vi "Python.vi"() -> ()   [LabVIEW 2014]
uses:
  Controls/Standard Action.ctl
  Controls/StageStates.ctl
  <vilib>/Analysis/baseanly.llb/Mean (DBL).vi
  <vilib>/Analysis/NI_AALBase.lvlib
panel:
  out "queue":string
  out "standard output":string
  out "standard error":string
  out "DM1":dbl[][](graph)
  out "DM0":dbl[][](graph)
  out "Image 2":sgl[][](graph)
  in  "launch_python":bool
  in  "script name":string="sensorless.py"
  in  "arguments":string="--zmin 11 --zmax 12 --nm-maxfev 80 --runs 1 --modes4pi --aberration-rms 0.0 --metric metric_low_spatial_freq modal"
  in  "Run Python":bool
  in  "Exit":bool
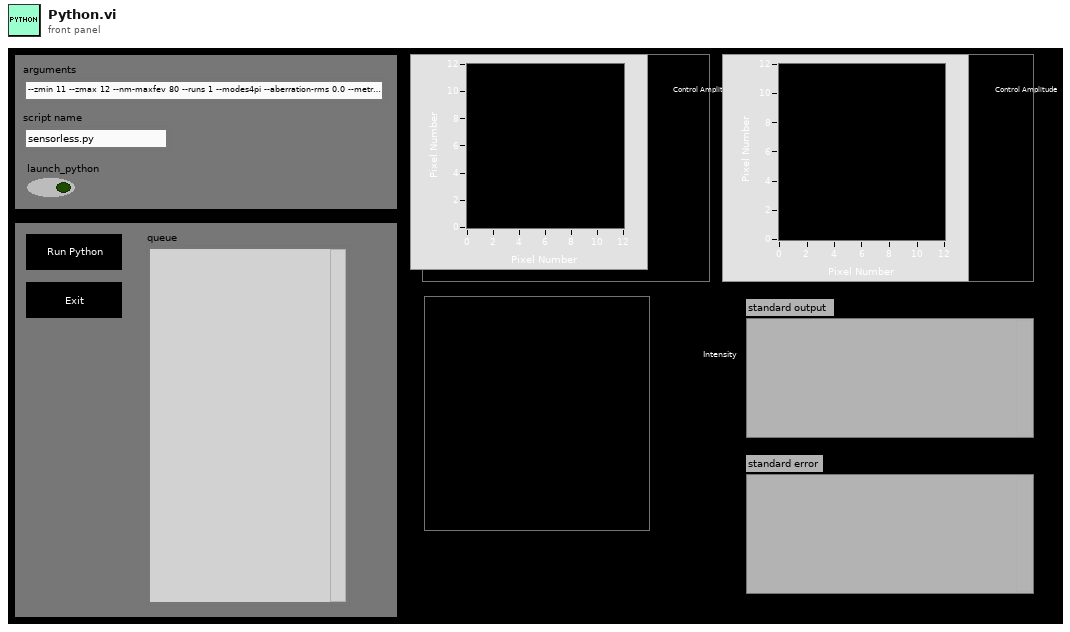
[diagram p1: front panel]
types:
  T1 = typedef "Standard Action.ctl" = enum16{"Read", "Write"}
  T2 = typedef "StageStates.ctl" = enum16{"POSITION", "MVR", "MOVE", "HALT", "ONTARGET", "ERROR", "EXIT", "HOME", "ZEROPOS", "NANOPOS", "QUIT", "ANALOG"}
  T3 = typedef "MirrorModes_DUAL.ctl" = cluster{"Mode":string, "Amplitude":dbl}[][]
  T4 = typedef "Image Acquisition Parameters.ctl" = cluster{"Scan Type":enum16{"Sample Scanning", "Beam Scanning"}, "Scan Mode":enum16{"XY", "XZ", "YZ", "XYZ"}, "Fast Axis Frequency (Hz)":dbl, "Image Format":u16, "Line Accumulations":u16, "Frames Per Capture":u16, "Frames Accumulations":u16, "Image Dimension (um)":dbl[], "Number of Z Steps":u16, "Z Steps Size (um)":dbl, "Pixel Size (nm)":dbl[], "Customized Image Format":dbl[]}
  T5 = typedef "Detectors.ctl" = cluster{"PMT":bool, "Far Red (685/40 nm)":bool, "Orange (624/40 nm)":bool, "Green (525/50 nm)":bool, "Sum All":bool}
  T6 = typedef "Laser Controls.ctl" = cluster{"STED Power (V)":dbl, "STED":bool, "650 nm":bool, "590 nm":bool, "485 nm":bool, "Manual Control":bool}
  T7 = cluster{"dm0":dbl[], "dm1":dbl[], "zcomp":dbl, "stack":sgl[][]}
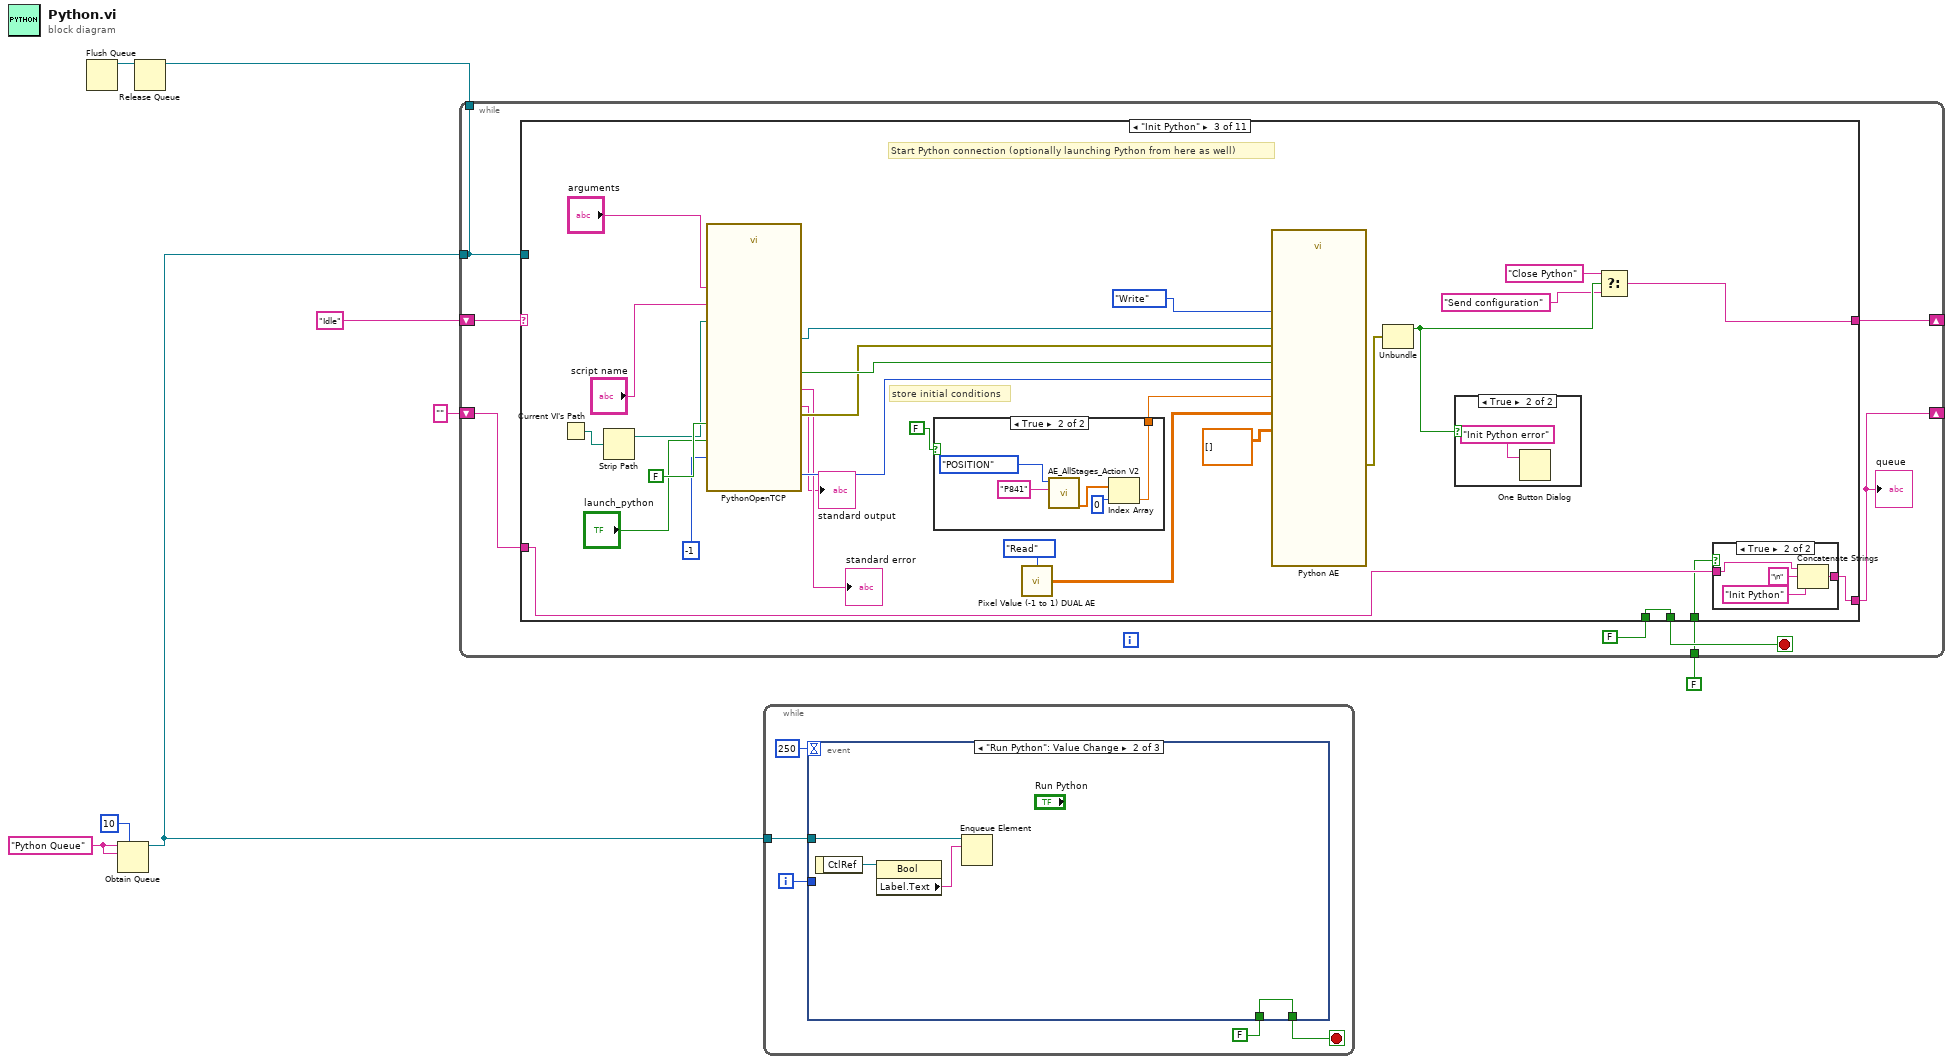
[diagram p0: block diagram]
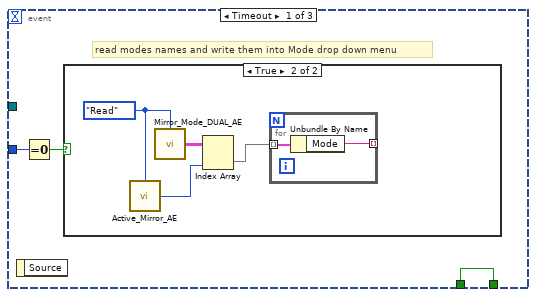
[diagram p2: hidden frame]
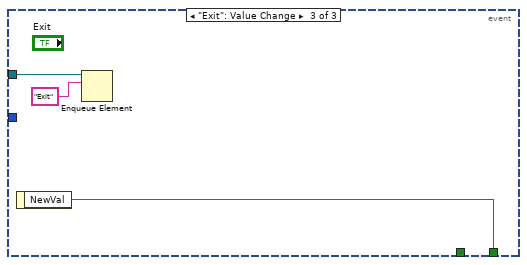
[diagram p4: hidden frame]
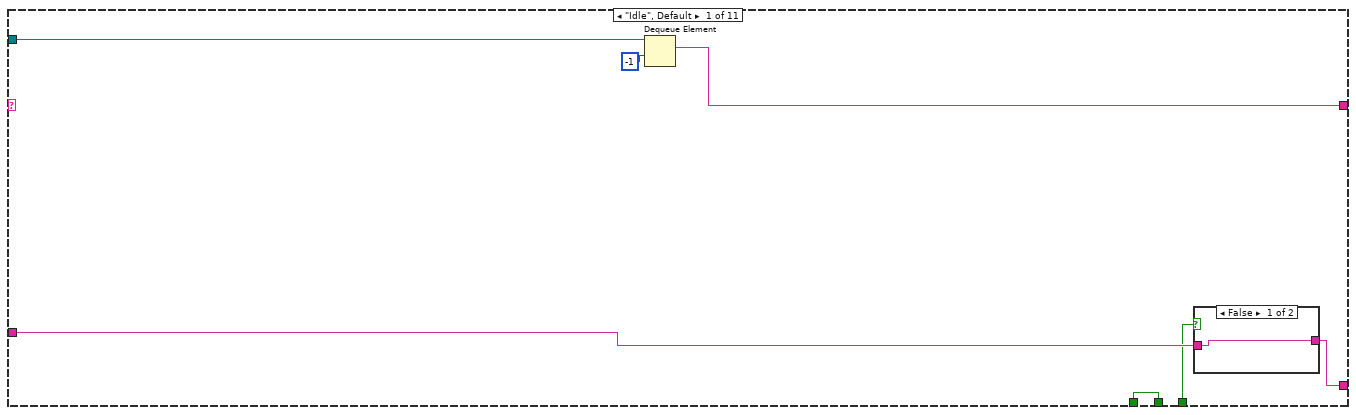
[diagram p5: hidden frame]
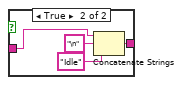
[diagram p6: hidden frame]
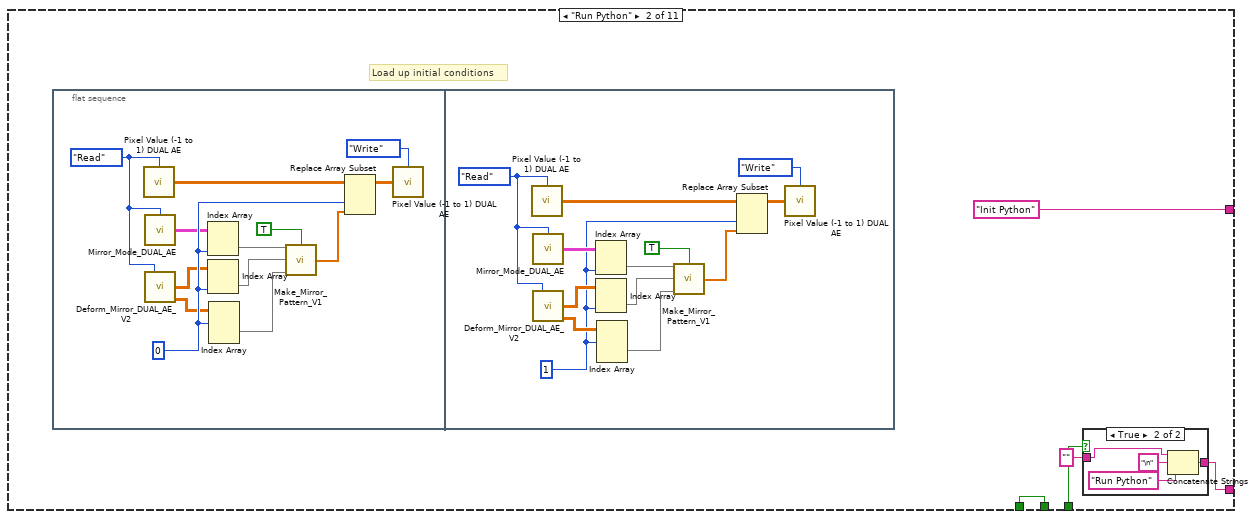
[diagram p7: hidden frame]
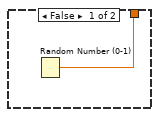
[diagram p10: hidden frame]
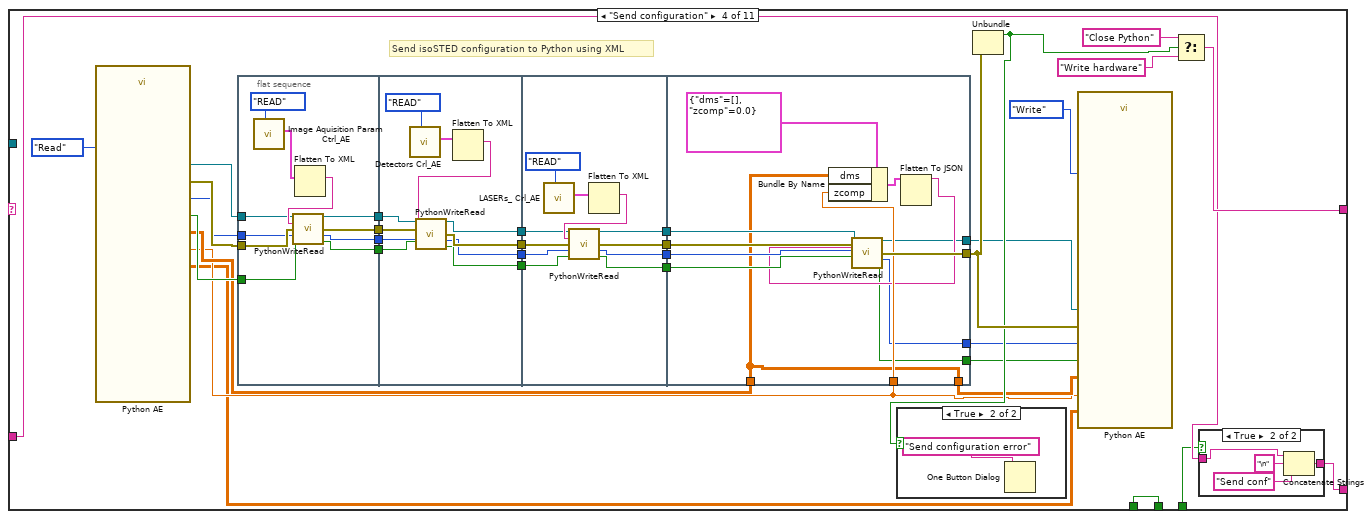
[diagram p12: hidden frame]
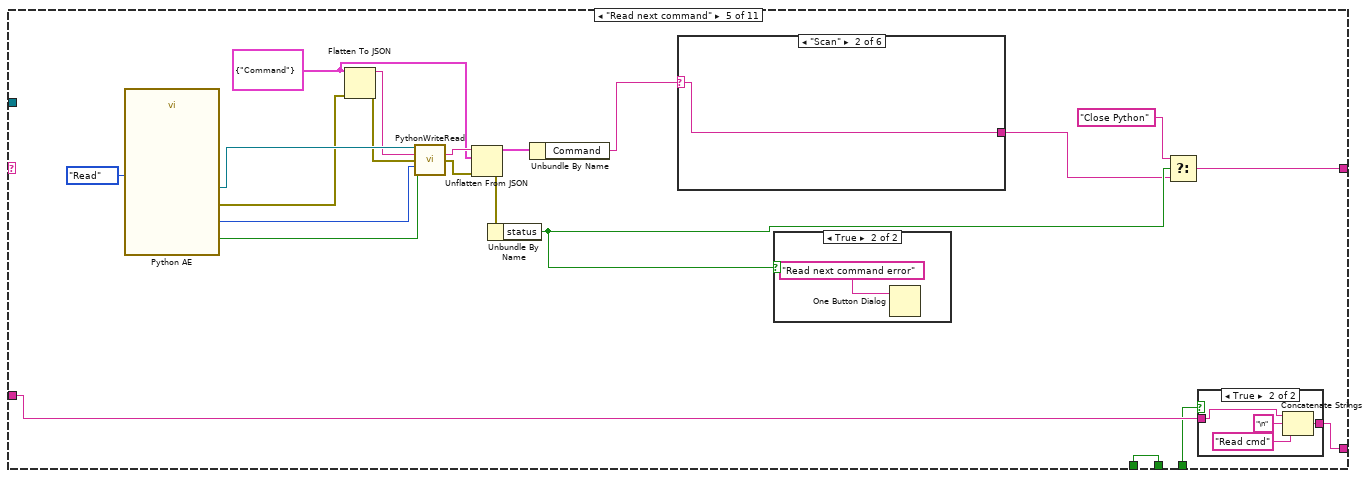
[diagram p15: hidden frame]
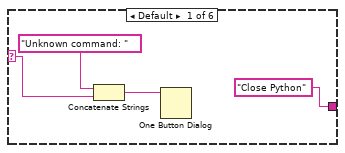
[diagram p17: hidden frame]
diagram:
  w7 = "Python Queue" ("name (unnamed)")
  n1 = Obtain Queue(max queue size (-1, unlimited)=10, name (unnamed)=w7, element data type=w7) -> (queue out=w5:refnum<queue>)  [unwired: 2 in, 2 out]
  n2 = while {
    shift-right: [w11] -> _
    shift-left: "Idle" -> [w13]
    tunnel: w5 -> [w15]
    tunnel: [w15] -> w4
    shift-right: [w10] -> _
    shift-left: "" -> [w12]
    tunnel: FALSE -> [w9]
    stop <- w16 stop-if-true
    n3 = case shown="\"Init Python\"" w13 {
      tunnel: [w20 w33 w82 w119 w210 w247 w270 w331 w364 w433 TRUE] -> w16
      tunnel: w15 -> [w22 _ _ _ _ _ _ _ _ _ _]
      tunnel: [w21 "Init Python" ("name (unnamed)") w70 w116 w195 w231 "Python pipe" ("name (unnamed)") w332 "Read next command" ("name (unnamed)") "Idle" ("name (unnamed)") "Exit" ("name (unnamed)")] -> w11
      tunnel: FALSE -> [w20 w33 w82 w119 w210 w247 w270 w331 w364 w433 _]
      tunnel: w12 -> [w19 _ w67 w107 w193 w228 w254 w318 w357 w420 w441]
      tunnel: [w17 w31 w66 w106 w192 w229 w256 w319 w356 w419 w442] -> w10
      tunnel: w9 -> [w18 w30 w65 w105 w191 w227 w255 w317 w358 w418 w440]
      frame "Idle", Default {
        n4 = Dequeue Element(queue=w22, timeout in ms (-1)=-1) -> (element=w21:string)  [unwired: 1 in, 3 out]
        n5 = case shown="False" w18 {
          tunnel: [w24 w26] -> w17
          tunnel: w19 -> [w24 w25]
          frame False {
          }
          frame True {
            n6 = Concatenate Strings(w25, "\n" ("string"), "Idle" ("string")) -> (w26:string)
          }
        }
      }
      frame "Run Python" {
        # "Load up initial conditions"
        n7 = flat-sequence {
          frame #0 {
            w51 = 0 ("index (col)")
            w47 = Standard_Action."Read" ("Action")
            n8 = call "Pixel Value (-1 to 1) DUAL AE.vi"("Action"=w47) -> ("Pixel Value (-1 to 1) Out"=w48:dbl[][])  [unwired: 14 in]
            n9 = call "Mirror_Mode_DUAL_AE.vi"("Action"=w47) -> ("Mirror Modes Out"=w44:T3)  [unwired: 14 in]
            n10 = call "Deform_Mirror_DUAL_AE_V2.vi"("Action"=w47) -> ("Flat Files Out"=w42:dbl[][], "Mode Matrix Out"=w40:dbl[][][])  [unwired: 10 in, 3 out]
            n11 = Index Array(array=w44, index (col)=w51) -> (element=w45:cluster{"Mode":string, "Amplitude":dbl}[])  [unwired: 1 in]
            n12 = Index Array(array=w42, index (col)=w51) -> (element=w43:dbl[])  [unwired: 1 in]
            n13 = Index Array(array=w40, index (dim 0)=w51) -> (element=w39:dbl[][])  [unwired: 2 in]
            n14 = call "Make_Mirror_Pattern_V1.vi"("Mirror Modes In"=w45, "Flat On?"=TRUE ("Apply Flat"), "Flat File In"=w43, "Mirror Modes Array"=w39) -> ("Pixel Value U (-1 to 1)"=w49:dbl[])  [unwired: 11 in]
            n15 = Replace Array Subset(array=w48, new element=w49, index (col)=w51) -> (w50:dbl[][])  [unwired: 1 in]
            n16 = call "Pixel Value (-1 to 1) DUAL AE.vi"("Action"=Standard_Action."Write", "Pixel Value (-1 to 1)"=w50) -> ()  [unwired: 13 in, 1 out]
          }
          frame #1 {
            w52 = 1 ("index (col)")
            w56 = Standard_Action."Read" ("Action")
            n17 = call "Pixel Value (-1 to 1) DUAL AE.vi"("Action"=w56) -> ("Pixel Value (-1 to 1) Out"=w55:dbl[][])  [unwired: 14 in]
            n18 = call "Mirror_Mode_DUAL_AE.vi"("Action"=w56) -> ("Mirror Modes Out"=w59:T3)  [unwired: 14 in]
            n19 = call "Deform_Mirror_DUAL_AE_V2.vi"("Action"=w56) -> ("Flat Files Out"=w61:dbl[][], "Mode Matrix Out"=w63:dbl[][][])  [unwired: 10 in, 3 out]
            n20 = Index Array(array=w59, index (col)=w52) -> (element=w58:cluster{"Mode":string, "Amplitude":dbl}[])  [unwired: 1 in]
            n21 = Index Array(array=w61, index (col)=w52) -> (element=w60:dbl[])  [unwired: 1 in]
            n22 = Index Array(array=w63, index (dim 0)=w52) -> (element=w64:dbl[][])  [unwired: 2 in]
            n23 = call "Make_Mirror_Pattern_V1.vi"("Mirror Modes In"=w58, "Flat On?"=TRUE ("Apply Flat"), "Flat File In"=w60, "Mirror Modes Array"=w64) -> ("Pixel Value U (-1 to 1)"=w54:dbl[])  [unwired: 11 in]
            n24 = Replace Array Subset(array=w55, new element=w54, index (col)=w52) -> (w53:dbl[][])  [unwired: 1 in]
            n25 = call "Pixel Value (-1 to 1) DUAL AE.vi"("Action"=Standard_Action."Write", "Pixel Value (-1 to 1)"=w53) -> ()  [unwired: 13 in, 1 out]
          }
        }
        n26 = case shown="True" w30 {
          tunnel: [w34 w36] -> w31
          tunnel: "" -> [w34 w35]
          frame False {
          }
          frame True {
            n27 = Concatenate Strings(w35, "\n" ("string"), "Run Python" ("string")) -> (w36:string)
          }
        }
      }
      frame "Init Python" {
        # "store initial conditions"
        # "Start Python connection (optionally launching Python from here as well)"
        n28 = Current VI's Path() -> (path=w74:path)
        n29 = Strip Path(path=w74) -> (stripped path=w73:path)  [unwired: 1 out]
        n30 = call "PythonOpenTCP.vi"("directory"=w73, "debug"=FALSE, "script name"="script name", "launch_python"="launch_python", "timeout in"=-1 ("timeout ms (60000)"), "arguments"="arguments") -> ("error out"=w83:errorcluster, "connection out"=w86:refnum<k5>, "standard error"=→"standard error":string, "timeout out"=w84:i32, "run_tcp"=w85:bool, "standard output"=→"standard output":string)  [unwired: 4 in]
        n31 = case shown="True" FALSE {
          tunnel: [w98 w99] -> w77
          frame False {
            n32 = Random Number (0-1)() -> (number: 0 to 1=w98:dbl)
          }
          frame True {
            n33 = call "AE_AllStages_Action V2.vi"("Stage ID"="P841" ("StageID"), "Action"=StageStates."POSITION") -> ("Position Out"=w102:dbl[])  [unwired: 7 in, 2 out]
            n34 = Index Array(array=w102, index=0) -> (element=w99:dbl)
          }
        }
        n35 = call "Pixel Value (-1 to 1) DUAL AE.vi"("Action"=Standard_Action."Read") -> ("Pixel Value (-1 to 1) Out"=w80:dbl[][])  [unwired: 14 in]
        n36 = call "Python AE.vi"("connection"=w86, "error"=w83, "run_tcp"=w85, "timeout"=w84, "u"=w80, "zcomp"=w77, "Action"=Standard_Action."Write", "stack"=sgl[][] []) -> ("error out"=w79:errorcluster)  [unwired: 5 in, 6 out]
        n37 = Unbundle(w79) -> ("status"=w72:bool)  [unwired: 2 out]
        n38 = case shown="True" w72 {
          frame False {
          }
          frame True {
            n39 = One Button Dialog(message="Init Python error") -> ()  [unwired: 1 in, 1 out]
          }
        }
        n40 = Select(t="Close Python", s=w72, f="Send configuration" ("name (unnamed)")) -> (s? t:f=w70:string)
        n41 = case shown="True" w65 {
          tunnel: [w93 w95] -> w66
          tunnel: w67 -> [w93 w94]
          frame False {
          }
          frame True {
            n42 = Concatenate Strings(w94, "\n" ("string"), "Init Python" ("string")) -> (w95:string)
          }
        }
      }
      frame "Send configuration" {
        # "Send isoSTED configuration to Python using XML"
        n43 = call "Python AE.vi"("Action"=Standard_Action."Read") -> ("zcomp out"=w109:dbl, "stack out"=w108:sgl[][], "connection out"=w125:refnum<k5>, "error out"=w124:errorcluster, "u out"=w111:dbl[][], "run_tcp out"=w122:bool, "timeout out"=w123:i32)  [unwired: 12 in]
        n44 = flat-sequence {
          tunnel: [w152] -> w138
          tunnel: [w151] -> w137
          tunnel: [w150] -> w136
          tunnel: [w149] -> w135
          tunnel: w125 -> [w148]
          tunnel: w124 -> [w147]
          tunnel: w123 -> [w146]
          tunnel: w122 -> [w145]
          tunnel: w138 -> [w163]
          tunnel: w137 -> [w162]
          tunnel: w136 -> [w161]
          tunnel: w135 -> [w160]
          tunnel: [w159] -> w134
          tunnel: [w158] -> w133
          tunnel: [w157] -> w132
          tunnel: [w156] -> w131
          tunnel: w134 -> [w174]
          tunnel: w133 -> [w173]
          tunnel: w132 -> [w172]
          tunnel: w131 -> [w171]
          tunnel: [w170] -> w130
          tunnel: [w169] -> w129
          tunnel: [w168] -> w128
          tunnel: [w167] -> w127
          tunnel: w130 -> [w189]
          tunnel: w129 -> [w188]
          tunnel: w128 -> [w187]
          tunnel: w127 -> [w186]
          tunnel: [w185] -> w120
          tunnel: w111 -> [w178]
          tunnel: w109 -> [w184]
          tunnel: [w181] -> w114
          tunnel: [w180] -> w113
          tunnel: [w179] -> w112
          tunnel: [w178] -> w110
          frame #0 {
            n45 = call "Image Aquisition Param Ctrl_AE.vi"("Action"=enum16{"READ", "WRITE"}."READ") -> ("Image Acquisition Parameters Out"=w155:T4)  [unwired: 10 in]
            n46 = Flatten To XML(anything=w155) -> (xml string=w153:string)
            n47 = call "PythonWriteRead.vi"("connection in"=w148, "string in"=w153, "error in"=w147, "timeout in"=w146, "run_tcp in"=w145) -> ("connection out"=w152:refnum<k5>, "error out"=w151:errorcluster, "timeout out"=w150:i32, "run_tcp out"=w149:bool)  [unwired: 6 in, 1 out]
          }
          frame #1 {
            n48 = call "Detectors Crl_AE.vi"("Action"=enum16{"READ", "WRITE"}."READ") -> ("Detectors Parameters Out"=w165:T5)  [unwired: 10 in]
            n49 = Flatten To XML(anything=w165) -> (xml string=w164:string)
            n50 = call "PythonWriteRead.vi"("connection in"=w163, "string in"=w164, "error in"=w162, "timeout in"=w161, "run_tcp in"=w160) -> ("connection out"=w159:refnum<k5>, "error out"=w158:errorcluster, "timeout out"=w157:i32, "run_tcp out"=w156:bool)  [unwired: 6 in, 1 out]
          }
          frame #2 {
            n51 = call "LASERs_ Crl_AE.vi"("Action"=enum16{"READ", "WRITE"}."READ") -> ("Laser Parameters Out"=w177:T6)  [unwired: 10 in]
            n52 = Flatten To XML(anything=w177) -> (xml string=w175:string)
            n53 = call "PythonWriteRead.vi"("connection in"=w174, "string in"=w175, "error in"=w173, "timeout in"=w172, "run_tcp in"=w171) -> ("connection out"=w170:refnum<k5>, "error out"=w169:errorcluster, "timeout out"=w168:i32, "run_tcp out"=w167:bool)  [unwired: 6 in, 1 out]
          }
          frame #3 {
            n54 = Bundle By Name(cluster=cluster{"dms":dbl[][], "zcomp":dbl} {"dms"=[], "zcomp"=0.0} ("input cluster"), "dms"=w178, "zcomp"=w184) -> (w183:cluster{"dms":dbl[][], "zcomp":dbl})
            n55 = Flatten To JSON(anything=w183) -> (JSON string=w182:string)  [unwired: 2 in, 1 out]
            n56 = call "PythonWriteRead.vi"("connection in"=w189, "string in"=w182, "error in"=w188, "timeout in"=w187, "run_tcp in"=w186) -> ("connection out"=w181:refnum<k5>, "error out"=w185:errorcluster, "timeout out"=w180:i32, "run_tcp out"=w179:bool)  [unwired: 6 in, 1 out]
          }
        }
        n57 = Unbundle(w120) -> ("status"=w115:bool)  [unwired: 2 out]
        n58 = case shown="True" w115 {
          frame False {
          }
          frame True {
            n59 = One Button Dialog(message="Send configuration error") -> ()  [unwired: 1 in, 1 out]
          }
        }
        n60 = call "Python AE.vi"("connection"=w114, "error"=w120, "run_tcp"=w112, "timeout"=w113, "u"=w110, "zcomp"=w109, "Action"=Standard_Action."Write", "stack"=w108) -> ()  [unwired: 5 in, 7 out]
        n61 = Select(t="Close Python", s=w115, f="Write hardware" ("name (unnamed)")) -> (s? t:f=w116:string)
        n62 = case shown="True" w105 {
          tunnel: [w139 w141] -> w106
          tunnel: w107 -> [w139 w140]
          frame False {
          }
          frame True {
            n63 = Concatenate Strings(w140, "\n" ("string"), "Send conf" ("string")) -> (w141:string)
          }
        }
      }
      frame "Read next command" {
        w202 = cluster{"Command":string} {"Command"="Command"} ("input cluster")
        n64 = call "Python AE.vi"("Action"=Standard_Action."Read") -> ("connection out"=w209:refnum<k5>, "error out"=w207:errorcluster, "run_tcp out"=w204:bool, "timeout out"=w205:i32)  [unwired: 12 in, 3 out]
        n65 = Flatten To JSON(anything=w202, error in (no error)=w207) -> (JSON string=w208:string, 11:w206:errorcluster)  [unwired: 1 in]
        n66 = call "PythonWriteRead.vi"("connection in"=w209, "string in"=w208, "error in"=w206, "timeout in"=w205, "run_tcp in"=w204) -> ("string out"=w203:string, "error out"=w201:errorcluster)  [unwired: 6 in, 3 out]
        n67 = Unflatten From JSON(JSON string=w203, type and defaults=w202, error in (no error)=w201) -> (value=w194:cluster{"Command":string}, error out=w200:errorcluster)  [unwired: 4 in]
        n68 = Unbundle By Name(w200) -> ("status"=w198:bool)
        n69 = Unbundle By Name(w194) -> ("Command"=w199:string)
        n70 = case shown="\"Scan\"" w199 {
          selector: w199 -> [w217 w221 w222 w223 w224 _]
          tunnel: ["Close Python" ("t") w221 w222 w223 w224 "Close Python" ("t")] -> w196
          frame Default {
            n71 = Concatenate Strings("Unknown command: " ("message"), w217) -> (w219:string)
            n72 = One Button Dialog(message=w219) -> ()  [unwired: 1 in, 1 out]
          }
          frame "Scan" {
          }
          frame "Image acquisition params" {
          }
          frame "Detectors params" {
          }
          frame "Laser params" {
          }
          frame "Stop" {
          }
        }
        n73 = case shown="True" w198 {
          frame False {
          }
          frame True {
            n74 = One Button Dialog(message="Read next command error") -> ()  [unwired: 1 in, 1 out]
          }
        }
        n75 = Select(t="Close Python" ("f"), s=w198, f=w196) -> (s? t:f=w195:string)
        n76 = case shown="True" w191 {
          tunnel: [w212 w214] -> w192
          tunnel: w193 -> [w212 w213]
          frame False {
          }
          frame True {
            n77 = Concatenate Strings(w213, "\n" ("string"), "Read cmd" ("string")) -> (w214:string)
          }
        }
      }
      frame "Image acquisition params" {
        # "Send isoSTED configuration to Python using XML"
        n78 = call "Python AE.vi"("Action"=Standard_Action."Read") -> ("connection out"=w245:refnum<k5>, "error out"=w244:errorcluster, "run_tcp out"=w242:bool, "timeout out"=w243:i32)  [unwired: 12 in, 3 out]
        n79 = call "Image Aquisition Param Ctrl_AE.vi"("Action"=enum16{"READ", "WRITE"}."READ") -> ("Image Acquisition Parameters Out"=w239:T4)  [unwired: 10 in]
        n80 = Flatten To XML(anything=w239) -> (xml string=w236:string)
        n81 = call "PythonWriteRead.vi"("connection in"=w245, "string in"=w236, "error in"=w244, "timeout in"=w243, "run_tcp in"=w242) -> ("string out"=w241:string, "error out"=w240:errorcluster)  [unwired: 6 in, 3 out]
        n82 = Unflatten From XML(xml string=w241, type=w239, error in (no error)=w240) -> (value=w234:T4, error out=w238:errorcluster)
        n83 = call "Image Aquisition Param Ctrl_AE.vi"("Action"=enum16{"READ", "WRITE"}."WRITE", "Image Acquisition Parameters In"=w234) -> ()  [unwired: 9 in, 1 out]
        n84 = Unbundle(w238) -> ("status"=w230:bool)  [unwired: 2 out]
        n85 = case shown="True" w230 {
          frame False {
          }
          frame True {
            n86 = One Button Dialog(message="Image acquisition params error") -> ()  [unwired: 1 in, 1 out]
          }
        }
        n87 = Select(t="Close Python", s=w230, f="Read next command" ("name (unnamed)")) -> (s? t:f=w231:string)
        n88 = case shown="True" w227 {
          tunnel: [w248 w250] -> w229
          tunnel: w228 -> [w248 w249]
          frame False {
          }
          frame True {
            n89 = Concatenate Strings(w249, "\n" ("string"), "Acq params" ("string")) -> (w250:string)
          }
        }
      }
      frame "Scan" {
        w275 = "Acquisition" ("name (unnamed)")
        # "Perform scan"
        n90 = Obtain Queue(max queue size (-1, unlimited)=10, name (unnamed)=w275, element data type=w275) -> (queue out=w272:refnum<queue>, created new?=w278:bool)  [unwired: 2 in, 1 out]
        n91 = Obtain Notifier(name (unnamed)="Running", notification data type=TRUE) -> (notifier out=w273:refnum<notifier>, created new?=w279:bool)  [unwired: 2 in, 1 out]
        n92 = Or(x=w278, y=w279) -> (x .or. y?=w280:bool)
        n93 = call "AE_AllStages_Action V2.vi"("Stage ID"="P841" ("StageID"), "Action"=StageStates."POSITION") -> ("Position Out"=w267:dbl[])  [unwired: 7 in, 2 out]
        n94 = case shown="False" w280 {
          tunnel: w272 -> [w289 _]
          tunnel: w273 -> [w287 _]
          tunnel: [w286 sgl[][] [] ("Value")] -> w258
          frame False {
            n95 = call "Graph Ref AE.vi"("Action"=enum16{"READ", "WRITE"}."READ") -> ("Graph Ref Out"=w297:refnum<vi>[])  [unwired: 10 in]
            n96 = Send Notification(notification=FALSE, notifier=w287) -> (notifier out=w292:refnum<notifier>, error out=w291:errorcluster)  [unwired: 1 in]
            n97 = Enqueue Element(queue=w289, element="Capture", error in (no error)=w291) -> (queue out=w293:refnum<queue>)  [unwired: 1 in, 2 out]
            n98 = Index Array(array=w297, index=0) -> (element=w299:refnum<vi>)
            n99 = while {
              tunnel: w292 -> [w305]
              tunnel: [w303] -> w294
              tunnel: w293 -> [w303]
              tunnel: [w302] -> w300
              tunnel: w299 -> [w302]
              stop <- w304 stop-if-true
              n100 = Get Notifier Status(notifier=w305) -> (current notification=w304:bool)  [unwired: 1 in, 4 out]
              n101 = Wait (ms)(milliseconds to wait=u32 100) -> ()  [unwired: 1 out]
            }
            n102 = property class="IntGraph (strict)"(reference=w300) -> ("Value"=w286:sgl[][])  [unwired: 1 in, 2 out]
            "Image 2" <- w286
            n103 = Enqueue Element(queue=w294, element="Stop Acquisition" ("f")) -> ()  [unwired: 2 in, 3 out]
          }
          frame True {
            # "Acquisition and Running were not found"
            n104 = One Button Dialog(message="Acquisition queue Not Found") -> ()  [unwired: 1 in, 1 out]
          }
        }
        n105 = Index Array(array=w267, index=0) -> (element=w257:dbl)
        n106 = call "Python AE.vi"("Action"=Standard_Action."Read") -> ("connection out"=w263:refnum<k5>, "error out"=w262:errorcluster, "u out"=w259:dbl[][], "run_tcp out"=w260:bool, "timeout out"=w261:i32)  [unwired: 12 in, 2 out]
        n107 = call "Python AE.vi"("connection"=w263, "error"=w262, "run_tcp"=w260, "timeout"=w261, "u"=w259, "zcomp"=w257, "Action"=Standard_Action."Write", "stack"=w258) -> ()  [unwired: 5 in, 7 out]
        n108 = case shown="True" w255 {
          tunnel: [w281 w283] -> w256
          tunnel: w254 -> [w281 w282]
          frame False {
          }
          frame True {
            n109 = Concatenate Strings(w282, "\n" ("string"), "Scan" ("string")) -> (w283:string)
          }
        }
      }
      frame "Python pipe" {
        w344 = T7 {"dm0"=[], "dm1"=[], "zcomp"=0.0, "stack"=[]} ("input cluster")
        # "Pipe scan data to Python using JSON"
        n110 = call "Python AE.vi"("Action"=Standard_Action."Read") -> ("zcomp out"=w323:dbl, "stack out"=w322:sgl[][], "connection out"=w316:refnum<k5>, "error out"=w320:errorcluster, "u out"=w326:dbl[][], "run_tcp out"=w312:bool, "timeout out"=w314:i32)  [unwired: 12 in]
        n111 = Index Array(array=w326, index (col)=1 ("disabled index (col)")) -> (element=w324:dbl[])  [unwired: 1 in]
        n112 = Index Array(array=w326, index (col)=0 ("disabled index (col)")) -> (element=w325:dbl[])  [unwired: 1 in]
        n113 = Bundle By Name(cluster=w344, "dm0"=w325, "dm1"=w324, "zcomp"=w323, "stack"=w322) -> (w343:T7)
        n114 = Flatten To JSON(anything=w343, error in (no error)=w320) -> (JSON string=w339:string, 11:w338:errorcluster)  [unwired: 1 in]
        n115 = call "PythonWriteRead.vi"("connection in"=w316, "string in"=w339, "error in"=w338, "timeout in"=w314, "run_tcp in"=w312) -> ("connection out"=w315:refnum<k5>, "string out"=w337:string, "error out"=w345:errorcluster, "timeout out"=w313:i32, "run_tcp out"=w311:bool)  [unwired: 6 in]
        n116 = Unflatten From JSON(JSON string=w337, type and defaults=w344, error in (no error)=w345) -> (value=w342:T7, error out=w328:errorcluster)  [unwired: 4 in]
        n117 = Unbundle By Name(w342) -> ("dm0"=w336:dbl[], "dm1"=w335:dbl[], "zcomp"=w329:dbl, "stack"=w321:sgl[][])
        n118 = Unbundle By Name(w328) -> ("status"=w310:bool)
        n119 = Build Array(w336, w335) -> (w309:dbl[][])
        n120 = Transpose 2D Array(2D array=w309) -> (transposed array=w308:dbl[][])
        n121 = case shown="True" w310 {
          frame False {
          }
          frame True {
            n122 = One Button Dialog(message="Python pipe error") -> ()  [unwired: 1 in, 1 out]
          }
        }
        n123 = call "Python AE.vi"("connection"=w315, "error"=w328, "run_tcp"=w311, "timeout"=w313, "u"=w308, "zcomp"=w329, "Action"=Standard_Action."Write", "stack"=w321) -> ()  [unwired: 5 in, 7 out]
        n124 = Select(t="Close Python", s=w310, f="Write hardware") -> (s? t:f=w332:string)
        n125 = case shown="True" w317 {
          tunnel: [w346 w348] -> w319
          tunnel: w318 -> [w346 w347]
          frame False {
          }
          frame True {
            n126 = Concatenate Strings(w347, "\n" ("string"), "Pipe" ("string")) -> (w348:string)
          }
        }
      }
      frame "Write hardware" {
        w368 = 12 ("dimension size")
        w378 = 12 ("dimension size")
        # "Update hardware settings (DMs and zcomp)"
        # "insert void pixels at corners as mean values"
        n127 = call "Python AE.vi"("Action"=Standard_Action."Read") -> ("zcomp out"=w362:dbl, "u out"=w365:dbl[][])  [unwired: 12 in, 5 out]
        n128 = In Range and Coerce(upper limit=14.5, x=w362, lower limit=0.5) -> (coerced(x)=w361:dbl)  [unwired: 1 out]
        n129 = Build Array(w361) -> (w391:dbl[])
        n130 = call "AE_AllStages_Action V2.vi"("Positions"=w391, "Stage ID"="P841" ("StageID"), "Action"=StageStates."MOVE") -> ()  [unwired: 6 in, 3 out]
        n131 = call "Pixel Value (-1 to 1) DUAL AE.vi"("Action"=Standard_Action."Write", "Pixel Value (-1 to 1)"=w365) -> ()  [unwired: 13 in, 1 out]
        n132 = Index Array(array=w365, index (col)=1 ("disabled index (col)")) -> (element=w354:dbl[])  [unwired: 1 in]
        n133 = Index Array(array=w365, index (col)=0 ("disabled index (col)")) -> (element=w355:dbl[])  [unwired: 1 in]
        n134 = flat-sequence {
          tunnel: w365 -> [w403]
          tunnel: [w403] -> w389
          tunnel: w389 -> [w412]
          frame #0 {
            w402 = 0 ("disabled index (col)")
            n135 = Index Array(array=w403, index (col)=w402) -> (element=w401:dbl[])  [unwired: 1 in]
            n136 = call "PythonVoltage2Signal.vi"("Control Signal In (-1~1)"=w401, "DM #"=w402) -> ("Voltage Out (0~Max. Vol.)"=w400:dbl[])  [unwired: 1 in, 1 out]
            n137 = call "Deform_Mirror_DUAL_AE_V2.vi"("Action"=Standard_Action."Read") -> ("Refnum Out"=w408:refnum<k7>, "IDs Out"=w405:i32[], "Multi Map Data Out"=w407:i32[])  [unwired: 10 in, 2 out]
            n138 = Index Array(array=w405, index=w402) -> (element=w404:i32)
            n139 = call "WriteDM_V2.vi"("reference in"=w408, "nDevId"=w404, "MultiDM  Mapping"=w407, "Voltage Array in"=w400) -> ()  [unwired: 2 in, 2 out]
          }
          frame #1 {
            w411 = 1 ("disabled index (col)")
            n140 = Index Array(array=w412, index (col)=w411) -> (element=w410:dbl[])  [unwired: 1 in]
            n141 = call "Deform_Mirror_DUAL_AE_V2.vi"("Action"=Standard_Action."Read") -> ("Refnum Out"=w413:refnum<k7>, "IDs Out"=w416:i32[], "Multi Map Data Out"=w414:i32[])  [unwired: 10 in, 2 out]
            n142 = call "PythonVoltage2Signal.vi"("Control Signal In (-1~1)"=w410, "DM #"=w411) -> ("Voltage Out (0~Max. Vol.)"=w409:dbl[])  [unwired: 1 in, 1 out]
            n143 = Index Array(array=w416, index=w411) -> (element=w417:i32)
            n144 = call "WriteDM_V2.vi"("reference in"=w413, "nDevId"=w417, "MultiDM  Mapping"=w414, "Voltage Array in"=w409) -> ()  [unwired: 2 in, 2 out]
          }
        }
        n145 = call-poly <vilib>:"Mean.vi"("X"=w354) -> ("mean"=w352:dbl)  [unwired: 1 out]
        n146 = call-poly <vilib>:"Mean.vi"("X"=w355) -> ("mean"=w353:dbl)  [unwired: 1 out]
        n147 = Insert Into Array(array=w354, index=0, new element=w352) -> (w374:dbl[])
        n148 = Insert Into Array(array=w355, index=0, new element=w353) -> (w384:dbl[])
        n149 = Insert Into Array(array=w374, index=11, new element=w352) -> (w372:dbl[])
        n150 = Insert Into Array(array=w384, index=11, new element=w353) -> (w382:dbl[])
        n151 = Insert Into Array(array=w372, index=132, new element=w352) -> (w370:dbl[])
        n152 = Insert Into Array(array=w382, index=132, new element=w353) -> (w380:dbl[])
        n153 = Insert Into Array(array=w370, index=143, new element=w352) -> (w377:dbl[])
        n154 = Insert Into Array(array=w380, index=143, new element=w353) -> (w387:dbl[])
        n155 = Reshape Array(w377, w368, w368) -> (→"DM1":dbl[][])
        n156 = Reshape Array(w387, w378, w378) -> (→"DM0":dbl[][])
        n157 = Wait (ms)(milliseconds to wait=u32 50) -> ()  [unwired: 1 out]
        n158 = case shown="True" w358 {
          tunnel: [w395 w397] -> w356
          tunnel: w357 -> [w395 w396]
          frame False {
          }
          frame True {
            n159 = Concatenate Strings(w396, "\n" ("string"), "Write HW" ("string")) -> (w397:string)
          }
        }
      }
      frame "Close Python" {
        n160 = call "Python AE.vi"("Action"=Standard_Action."Read") -> ("connection out"=w431:refnum<k5>, "error out"=w429:errorcluster, "run_tcp out"=w430:bool)  [unwired: 12 in, 4 out]
        n161 = call "PythonCloseTCP.vi"("connection in"=w431, "run_tcp"=w430, "error in"=w429) -> ()  [unwired: 12 in, 1 out]
        n162 = call "Python AE.vi"("connection"=refnum<k5> refnum, "error"=errorcluster {"status"=FALSE, "code"=0, "source"=""}, "run_tcp"=FALSE, "timeout"=-1, "u"=dbl[][] [], "zcomp"=0.0, "Action"=Standard_Action."Write", "stack"=sgl[][] []) -> ()  [unwired: 5 in, 7 out]
        n163 = case shown="True" w418 {
          tunnel: [w435 w437] -> w419
          tunnel: w420 -> [w435 w436]
          frame False {
          }
          frame True {
            n164 = Concatenate Strings(w436, "\n" ("string"), "Close Python" ("string")) -> (w437:string)
          }
        }
      }
      frame "Exit" {
        n165 = case shown="True" w440 {
          tunnel: [w445 w447] -> w442
          tunnel: w441 -> [w445 w446]
          frame False {
          }
          frame True {
            n166 = Concatenate Strings(w446, "\n" ("string"), "Exit" ("string")) -> (w447:string)
          }
        }
      }
    }
    "queue" <- w10
  }
  n167 = Flush Queue(queue=w4) -> (queue out=w3:refnum<queue>)  [unwired: 1 in, 2 out]
  n168 = Release Queue(queue=w3) -> ()  [unwired: 2 in, 3 out]
  n169 = while {
    tunnel: w5 -> [w454]
    i -> [w451]
    stop <- w453 stop-if-true
    n170 = event shown="[1] \"Run Python\": Value Change" {
      selector: _ -> [_ _ _]
      dyn-events: _ -> [_ _ _]
      timeout: 250 -> [_ _ _]
      tunnel: w454 -> [_ w466 w470]
      tunnel: [w457 w464 w468] -> w453
      tunnel: FALSE -> [w457 w464 _]
      tunnel: w451 -> [w456 _ _]
      event Timeout {
        # "read modes names and write them into Mode drop down menu"
        n171 = event-data() -> ()  [unwired: 1 in, 1 out]
        n172 = Equal To 0?(x=w456) -> (x = 0?=w455:bool)
        n173 = case shown="True" w455 {
          frame False {
          }
          frame True {
            w461 = Standard_Action."Read" ("Action")
            n174 = call "Active_Mirror_AE.vi"("Action"=w461) -> ("Active Mirror"=w458:i32)  [unwired: 14 in]
            n175 = call "Mirror_Mode_DUAL_AE.vi"("Action"=w461) -> ("Mirror Modes Out"=w460:T3)  [unwired: 14 in]
            n176 = Index Array(array=w460, index (col)=w458) -> (element=w459:cluster{"Mode":string, "Amplitude":dbl}[])  [unwired: 1 in]
            n177 = for {
              tunnel: w459 -> [w463] mode=indexing
              tunnel: [w462] -> _ mode=indexing
              n178 = Unbundle By Name(w463) -> ("Mode"=w462:string)
            }
          }
        }
      }
      event "Run Python": Value Change {
        n179 = event-data() -> ("CtlRef"=w465:refnum<vi>)  [unwired: 1 in]
        n180 = property class="Bool"(reference=w465) -> ("Label.Text"=w467:string)  [unwired: 1 in, 2 out]
        n181 = Enqueue Element(queue=w466, element=w467) -> ()  [unwired: 2 in, 3 out]
      }
      event "Exit": Value Change {
        n182 = event-data() -> ("NewVal"=w468:bool)  [unwired: 1 in]
        n183 = Enqueue Element(queue=w470, element="Exit") -> ()  [unwired: 2 in, 3 out]
      }
    }
  }
